vi "user initialization.vi"(8 "error in":errorcluster, 10 "configuration in":refnum<class "control module configuration.lvclass">, 11 "fixed channel runtime in":refnum<class "ActiveFrontEndModule runtime.lvclass">) -> (0 "error out":errorcluster, 3 "fixed channel runtime out":refnum<class "ActiveFrontEndModule runtime.lvclass">)   [LabVIEW 2017, in "ActiveFrontEndModule runtime.lvclass"]
uses:
  ActiveFrontEndModule runtime.lvclass
  <vilib>/NI/DCAF/Tag Editor Core/control module/configuration/control module configuration.lvclass
  <vilib>/userdefined/High Color/nirio_resource_hc.ctl
  <vilib>/NI/DCAF/addons/InstructionFrameworkSupport/FPGA_FGV_action.ctl
  configuration/ActiveFrontEndModule configuration.lvclass
  C:/Program Files (x86)/National Instruments/LabVIEW 2017/vi.lib/NI/DCAF/Tag Editor Core/control module/configuration/control module configuration.lvclass
  <vilib>/NI/PowerElectronicsControl/ActiveFrontEnd/AFE_Interface/PI_Controllers.ctl
  configuration/ActiveFrontEndModule configuration.lvclass/ActiveFrontEndModule configuration.ctl
  configuration/Read Parameters.vi
  configuration/Read VDCLinkToPower.vi
  configuration/Read ID_to_VD.vi
  configuration/Read IQ_to_VQ.vi
  <instrlib>/_niInstr/FIFO Register Bus/v1/Host/niInstr FIFO Register Bus v1 Host.lvclass
  C:/Program Files (x86)/National Instruments/LabVIEW 2017/instr.lib/_niInstr/Instruction Framework/v1/Host/Instruction Target/niInstr Instruction Target v1 Host.lvclass
  <vilib>/NI/DCAF/Tag Editor Core/control module/runtime/control module runtime.lvclass
  <instrlib>/_niInstr/Instruction Framework/v1/Host/Subsystem Map/niInstr Subsystem Map v1 Host.lvclass
  <vilib>/NI/PowerElectronicsControl/ActiveFrontEnd/AFE_Interface/AFE_interface.lvlib
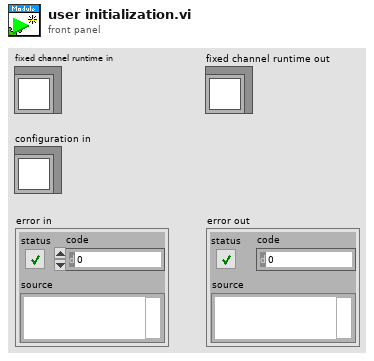
[diagram p1: front panel]
types:
  T1 = typedef "AFE_interface.lvlib/PI_Controllers.ctl" = enum16{"VDCLink to Power", "ID to VD", "IQ to VQ"}
  T2 = typedef "FPGA_FGV_action.ctl" = enum16{"get FPGA", "set FPGA", "Close"}
  T3 = typedef "nirio_resource_hc.ctl" = tag
  T4 = typedef "ActiveFrontEnd.lvlib/Parameters.ctl" = cluster{"VDCLink_setpt":sgl, "VDCLinkRampRate":sgl, "Q_setpt":sgl, "Pf_setpt":sgl, "Mode":T5, "perturbance_amp":sgl, "perturbance_freq":sgl, "dT":sgl}
  T5 = typedef "ActiveFrontEnd.lvlib/Mode.ctl" = enum16{"Q Control", "Pf Control"}
  T6 = typedef "ActiveFrontEnd.lvlib/PI_Settings.ctl" = cluster{"gains":T7, "output range":T8, "PI_state":enum8{"idle", "normal", "manual", "perturbance"}, "reset":bool, "manual":sgl}
  T7 = typedef "niFpgaPID_PIGains.ctl" = cluster{"proportional gain":sgl, "integral gain":sgl}
  T8 = typedef "niFpgaPID_OutputRange.ctl" = cluster{"output high (Inf)":sgl, "output low (-Inf)":sgl}
  T9 = typedef "AFE_interface.lvlib/InterfaceRef.ctl" = cluster{"instruction target":refnum<class "niInstr Instruction Target v1 Host.lvclass">, "context":refnum<class "niInstr Instruction Framework Context v1 Host.lvclass">}
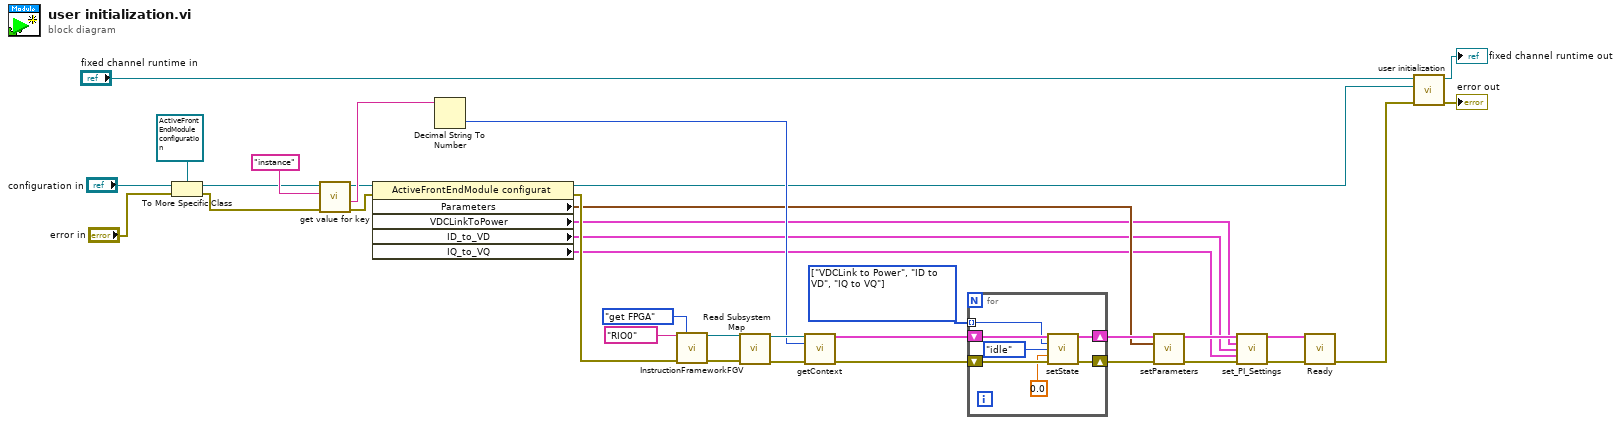
[diagram p0: block diagram]
diagram:
  w16 = T1[] [enum."VDCLink to Power", enum."ID to VD", enum."IQ to VQ"] items=["VDCLink to Power", "ID to VD", "IQ to VQ"]
  n1 = To More Specific Class(target class=refnum<class "ActiveFrontEndModule configuration.lvclass"> refnum ("ActiveFrontEndModule configuration"), reference="configuration in", error in="error in") -> (specific class reference=w26:refnum<class "ActiveFrontEndModule configuration.lvclass">, error out=w25:errorcluster)
  n2 = call-dynamic "get value for key.vi"("error in"=w25, "key"="instance", "fixed channel configuration in"=w26) -> ("error out"=w7:errorcluster, "value"=w21:string, "fixed channel configuration out"=w8:refnum<class "ActiveFrontEndModule configuration.lvclass">)  [unwired: 6 in]
  n3 = property class="ActiveFrontEndModule configurat"(reference=w8, error in=w7) -> (reference out=w5:refnum<class "ActiveFrontEndModule configuration.lvclass">, error out=w6:errorcluster, "Parameters"=w4:T4, "VDCLinkToPower"=w3:T6, "ID_to_VD"=w2:T6, "IQ_to_VQ"=w1:T6)
  n4 = Decimal String To Number(string=w21) -> (number=w20:i32)  [unwired: 2 in, 1 out]
  n5 = call <vilib>:"InstructionFrameworkFGV.vi"("RIO resource"=T3 "RIO0", "Action"=FPGA_FGV_action."get FPGA", "error in"=w6) -> ("session out"=w29:refnum<class "niInstr FIFO Register Bus v1 Host.lvclass">, "error out"=w30:errorcluster)  [unwired: 10 in, 1 out]
  n6 = call <instrlib>:"Read Subsystem Map.vi"("instruction target in"=w29, "error in"=w30) -> ("instruction target out"=w28:refnum<class "niInstr FIFO Register Bus v1 Host.lvclass">, "error out"=w19:errorcluster)  [unwired: 11 in, 1 out]
  n7 = call <vilib>:"getContext.vi"("instruction target in"=w28, "instance"=w20, "error in"=w19) -> ("Interface"=w18:T9, "error out"=w17:errorcluster)  [unwired: 11 in]
  n8 = for {
    shift-right: [w38] -> w15
    shift-left: w18 -> [w42]
    shift-right: [w37] -> w14
    shift-left: w17 -> [w41]
    tunnel: w16 -> [w36] mode=indexing
    n9 = call <vilib>:"setState.vi"("Interface in"=w42, "PI_Controller"=w36, "PI_state"=enum8{"idle", "normal", "manual", "perturbance"}."idle", "manual"=sgl 0.0, "error in"=w41) -> ("Interface out"=w38:T9, "error out"=w37:errorcluster)  [unwired: 9 in]
  }
  n10 = call <vilib>:"setParameters.vi"("Interface in"=w15, "Parameters"=w4, "error in"=w14) -> ("Interface out"=w13:T9, "error out"=w12:errorcluster)  [unwired: 11 in]
  n11 = call <vilib>:"set_PI_Settings.vi"("Interface in"=w13, "VDCLinkToPower"=w3, "ID_to_VD"=w2, "IQ_to_VQ"=w1, "error in"=w12) -> ("Interface out"=w10:T9, "error out"=w9:errorcluster)  [unwired: 9 in]
  n12 = call <vilib>:"Ready.vi"("Interface in"=w10, "error in"=w9) -> ("error out"=w11:errorcluster)  [unwired: 12 in, 1 out]
  n13 = call-parent "user initialization.vi"("error in"=w11, "configuration in"=w5, "fixed channel runtime in"="fixed channel runtime in") -> ("error out"=→"error out":errorcluster, "fixed channel runtime out"=→"fixed channel runtime out":refnum<class "ActiveFrontEndModule runtime.lvclass">)  [unwired: 7 in]
